vi "set_content_at.vi"(4 "value is XML itself?":bool, 5 "enforce empty content?":bool, 6 "id chain":string[](array[string]), 7 "attribute name":string, 8 "error in (no error)":errorcluster, 9 "content":string, 10 "key chain":string[](array[string]), 11 "Element in":refnum<class "XMLElement.lvclass">) -> (0 "error out":errorcluster, 3 "Element out":refnum<class "XMLElement.lvclass">)   [LabVIEW 2010, in "XMLElement.lvclass"]
uses:
  XMLElement.lvclass
  Program Files (x86)/National Instruments/LabVIEW 2010/resource/objmgr/DOMUserDefRef.rc
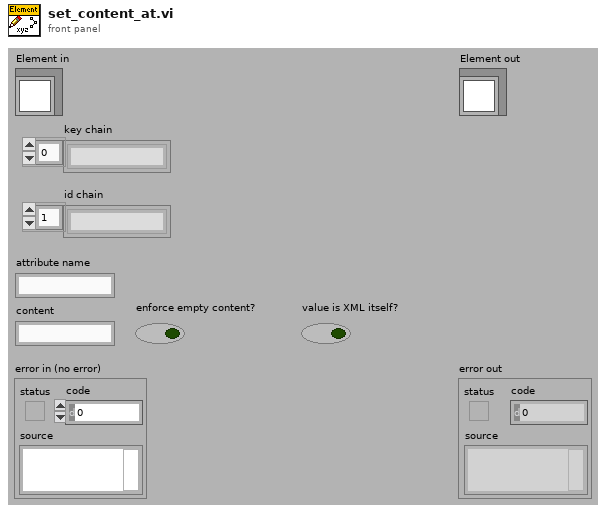
[diagram p1: front panel]
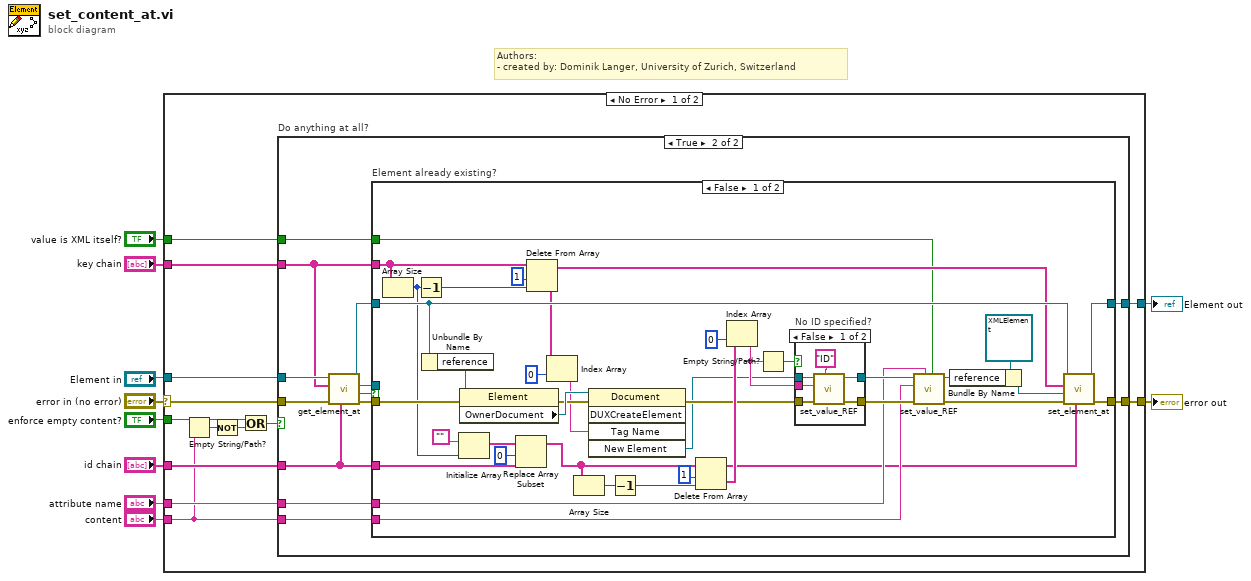
[diagram p0: block diagram]
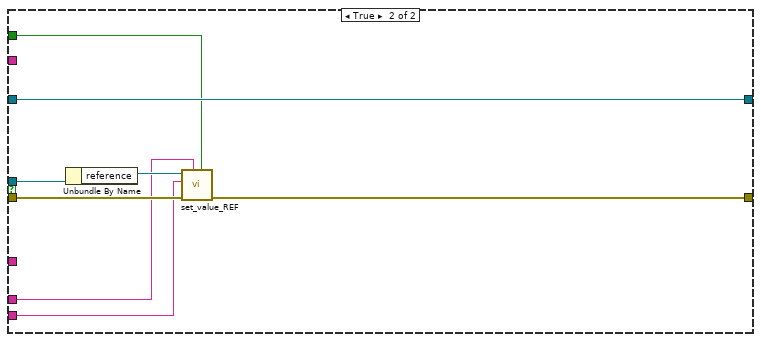
[diagram p4: hidden frame]
diagram:
  # "Authors: \n- created by: Dominik Langer, University of Zurich, Switzerland"
  n1 = case shown="No Error" "error in (no error)" {
    selector: "error in (no error)" -> [w20 w95]
    tunnel: [w23 w95] -> w9
    tunnel: [w22 w94] -> w7
    tunnel: "Element in" -> [w19 w94]
    tunnel: "key chain" -> [w18 _]
    tunnel: "id chain" -> [w17 _]
    tunnel: "attribute name" -> [w21 _]
    tunnel: "content" -> [w16 _]
    tunnel: "enforce empty content?" -> [w13 _]
    tunnel: "value is XML itself?" -> [w11 _]
    frame No Error {
      n2 = Empty String/Path?(string/path=w16) -> (empty?=w15:bool)
      n3 = Not(x=w15) -> (.not. x?=w14:bool)
      n4 = Or(x=w13, y=w14) -> (x .or. y?=w12:bool)
      n5 = case "Do anything at all?" shown="True" w12 {
        tunnel: [w25 w32] -> w23
        tunnel: [w24 w31] -> w22
        tunnel: w21 -> [_ w34]
        tunnel: w20 -> [w25 w38]
        tunnel: w19 -> [w24 w30]
        tunnel: w18 -> [_ w28]
        tunnel: w17 -> [_ w27]
        tunnel: w16 -> [_ w33]
        tunnel: w11 -> [_ w26]
        frame False {
        }
        frame True {
          n6 = call "get_element_at.vi"("id chain"=w27, "error in (no error)"=w38, "key chain"=w28, "Element in"=w30) -> ("error out"=w37:errorcluster, "found?"=w36:bool, "element"=w35:refnum<class "XMLElement.lvclass">, "Element out"=w29:refnum<class "XMLElement.lvclass">)  [unwired: 4 in]
          n7 = case "Element already existing?" shown="False" w36 {
            tunnel: w37 -> [w59 w91]
            tunnel: w35 -> [_ w93]
            tunnel: w34 -> [w47 w87]
            tunnel: w29 -> [w75 w92]
            tunnel: w33 -> [w48 w88]
            tunnel: [w77 w89] -> w32
            tunnel: [w76 w92] -> w31
            tunnel: w28 -> [w66 _]
            tunnel: w27 -> [w40 _]
            tunnel: w26 -> [w45 w86]
            frame False {
              n8 = Array Size(array=w66) -> (size(s)=w43:i32)
              n9 = Decrement(x=w43) -> (x-1=w65:i32)
              n10 = Unbundle By Name(w75) -> ("reference"=w58:refnum<k20>)
              n11 = Initialize Array("", w43) -> (w42:string[])
              n12 = property class="Element"(reference=w58, error in=w59) -> (error out=w71:errorcluster, "OwnerDocument"=w72:refnum<k20>)  [unwired: 1 out]
              n13 = Replace Array Subset(array=w42, new element=w40, index=0) -> (w39:string[])
              n14 = Delete From Array(array=w66, length=1, index=w65) -> (deleted portion=w63:string[], array with subset deleted=w64:string[])
              n15 = Index Array(array=w63, index=0) -> (element=w61:string)
              n16 = Array Size(array=w39) -> (size(s)=w68:i32)
              n17 = invoke class="Document" method="DUXCreateElement"(reference=w72, error in=w71, "Tag Name"=w61) -> (error out=w57:errorcluster, "New Element"=w50:refnum<k20>)  [unwired: 2 in, 3 out]
              n18 = Decrement(x=w68) -> (x-1=w67:i32)
              n19 = Delete From Array(array=w39, length=1, index=w67) -> (deleted portion=w60:string[], array with subset deleted=w46:string[])
              n20 = Index Array(array=w60, index=0) -> (element=w55:string)
              n21 = Empty String/Path?(string/path=w55) -> (empty?=w54:bool)
              n22 = case "No ID specified?" shown="False" w54 {
                tunnel: w50 -> [w80 w84]
                tunnel: w57 -> [w83 w85]
                tunnel: [w82 w85] -> w53
                tunnel: w55 -> [w78 _]
                tunnel: [w81 w84] -> w52
                frame False {
                  n23 = call "set_value_REF.vi"("attribute name"="ID" ("Name"), "error in (no error)"=w83, "value"=w78, "Element ref in"=w80) -> ("error out"=w82:errorcluster, "Element ref out"=w81:refnum<k20>)  [unwired: 6 in]
                }
                frame True {
                }
              }
              n24 = call "set_value_REF.vi"("treat value as XML?"=w45, "attribute name"=w47, "error in (no error)"=w53, "value"=w48, "Element ref in"=w52) -> ("error out"=w51:errorcluster, "Element ref out"=w49:refnum<k20>)  [unwired: 5 in]
              n25 = Bundle By Name(cluster=refnum<class "XMLElement.lvclass"> refnum ("XMLElement.lvclass"), "reference"=w49) -> (w73:refnum<class "XMLElement.lvclass">)
              n26 = call "set_element_at.vi"("id chain"=w46, "error in (no error)"=w51, "element"=w73, "key chain"=w64, "Element in"=w75) -> ("error out"=w77:errorcluster, "Element out"=w76:refnum<class "XMLElement.lvclass">)  [unwired: 5 in]
            }
            frame True {
              n27 = Unbundle By Name(w93) -> ("reference"=w90:refnum<k20>)
              n28 = call "set_value_REF.vi"("treat value as XML?"=w86, "attribute name"=w87, "error in (no error)"=w91, "value"=w88, "Element ref in"=w90) -> ("error out"=w89:errorcluster)  [unwired: 5 in, 1 out]
            }
          }
        }
      }
    }
    frame Error {
    }
  }
  "error out" <- w9
  "Element out" <- w7
